vi "GetNetworkInfo.vi"(8 "error in":errorcluster) -> (0 "error out":errorcluster, 2 "MAC Address":string, 3 "IP Address":string)   [LabVIEW 2014, in "hse-network.lvlib"]
doc: "(v0.2.1b; 2017-08-14 16:44)\n\n\n\n____\nHAMPEL SOFTWARE ENGINEERING v0.7.0 (2018-07-16 18:12)"
uses:
  hse-network.lvlib
  <resource>/objmgr/nisysapi.rc
  <vilib>/nisyscfg/nisyscfg.lvlib
  <vilib>/nisyscfg/Close (System).vi
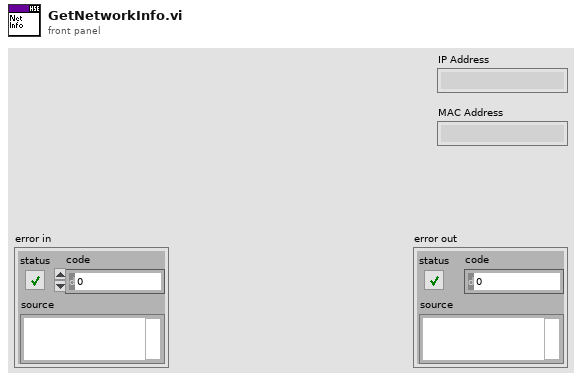
[diagram p1: front panel]
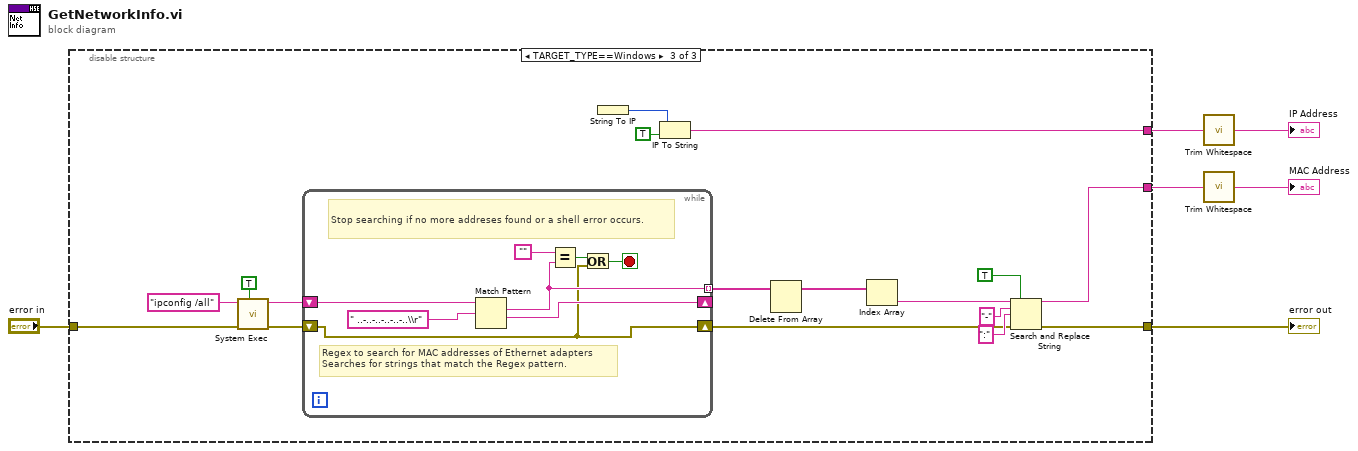
[diagram p0: block diagram]
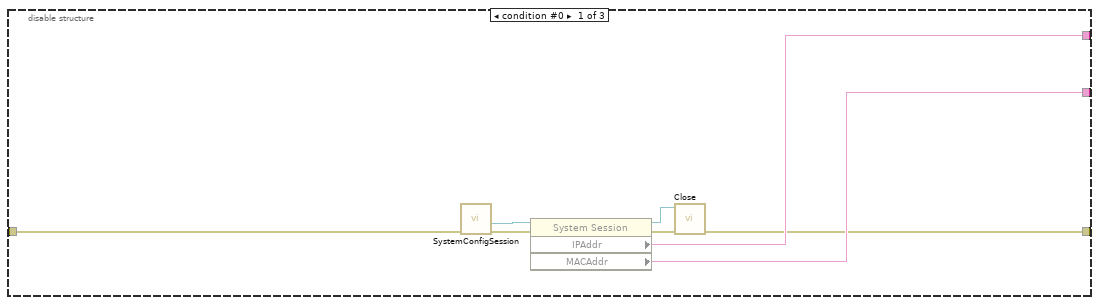
[diagram p2: hidden frame]
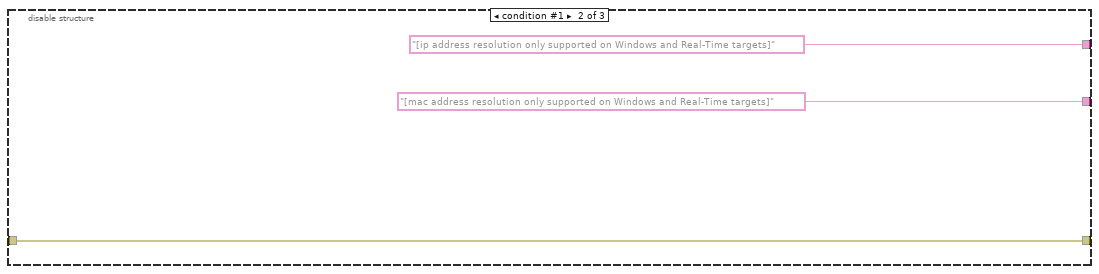
[diagram p3: hidden frame]
diagram:
  n1 = disable-structure shown="TARGET_TYPE==Windows" {
    disable-tunnel: [w14 "[mac address resolution only supported on Windows and Real-Time targets]" ("MACAddr") w23] -> w3
    disable-tunnel: [w13 "[ip address resolution only supported on Windows and Real-Time targets]" ("MACAddr") w25] -> w4
    disable-tunnel: "error in" -> [w9 w16 w28]
    disable-tunnel: [w10 w16 w18] -> w5
    frame condition #0 {
      n2 = call "SystemConfigSession.vi"("error in"=w9) -> ("error out"=w8:errorcluster, "Refnum out"=w7:refnum<k21>)  [unwired: 9 in]
      n3 = property class="System Session"(reference=w7, error in=w8) -> (reference out=w12:refnum<k21>, error out=w11:errorcluster, "IPAddr"=w13:string, "MACAddr"=w14:string)
      n4 = call-poly <vilib>:"Close.vi"("error in (no error)"=w11, "Session in"=w12) -> ("error out"=w10:errorcluster)  [unwired: 9 in]
    }
    frame condition #1 {
    }
    frame condition #2 (active) {
      n5 = call <vilib>:"System Exec.vi"("run minimized? (F)"=TRUE, "error in (no error)"=w28, "command line"="ipconfig /all") -> ("error out"=w33:errorcluster, "standard output"=w31:string)  [unwired: 5 in, 2 out]
      n6 = while {
        shift-right: [w40] -> _
        shift-left: w31 -> [w41]
        tunnel: [w39] -> w32 mode=indexing
        shift-right: [w35] -> w19
        shift-left: w33 -> [w35]
        stop <- w36 stop-if-true
        # "Stop searching if no more addreses found or a shell error occurs."
        # "Regex to search for MAC addresses of Ethernet adapters\nSearches for strings that match the Regex pattern."
        n7 = Match Pattern(string=w41, regular expression=" ..-..-..-..-..-..\\r") -> (match substring=w39:string, after substring=w40:string)  [unwired: 1 in, 2 out]
        n8 = Equal?(x="", y=w39) -> (x = y?=w37:bool)
        n9 = Or(x=w37, y=w35) -> (x .or. y?=w36:bool)
      }
      n10 = String To IP() -> (0:w26:u32)  [unwired: 1 in]
      n11 = IP To String(1:TRUE ("dot notation? (F)"), 2:w26) -> (0:w25:string)
      n12 = Delete From Array "Delete From Array"(array=w32) -> (array with subset deleted=w34:string[])  [unwired: 2 in, 1 out]
      n13 = Index Array "Index Array"(array=w34) -> (element=w24:string)  [unwired: 1 in]
      n14 = Search and Replace String(replace all?=TRUE ("replace all? (F)"), input string=w24, search string="-", replace string=":" ("replace string (\"\")"), error in=w19) -> (result string=w23:string, error out=w18:errorcluster)  [unwired: 3 in, 2 out]
    }
  }
  "error out" <- w5
  n15 = call <vilib>:"Trim Whitespace.vi"("string"=w4) -> ("trimmed string"=→"IP Address":string)  [unwired: 1 in]
  n16 = call <vilib>:"Trim Whitespace.vi"("string"=w3) -> ("trimmed string"=→"MAC Address":string)  [unwired: 1 in]
